vi "基恩士扫码枪.vi"(8 "error in":errorcluster) -> (0 "error out":errorcluster, 1 "扫码内容":string, 2 "扫码成功":bool)   [LabVIEW 2014]
uses:
  Controls/MsgAction.ctl
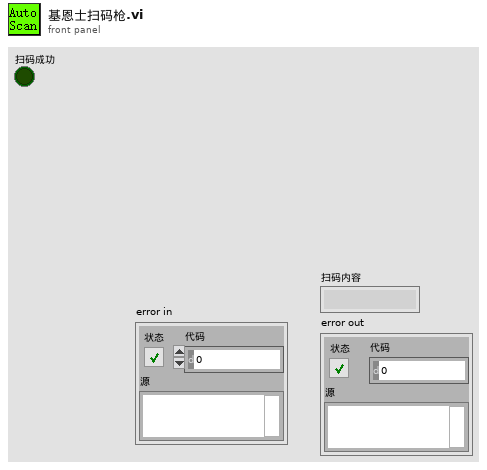
[diagram p1: front panel]
types:
  T1 = typedef "MsgAction.ctl" = enum16{"初始化", "添加消息", "区分结果添加消息", "清空消息", "获取消息"}
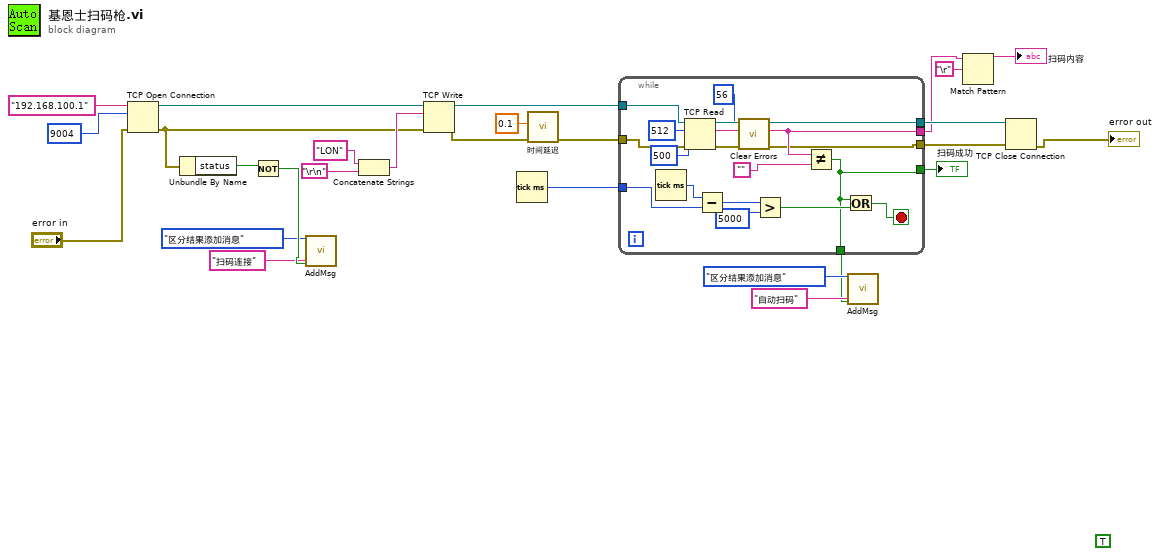
[diagram p0: block diagram]
diagram:
  (unwired) TRUE
  n1 = TCP Open Connection(address="192.168.100.1" ("地址"), remote port or service name=u16 9004 ("远程端口或服务名称"), error in (no error)="error in") -> (connection ID=w11:refnum<k5>, error out=w9:errorcluster)  [unwired: 2 in]
  n2 = Unbundle By Name(w9) -> ("status"=w26:bool)
  n3 = Not(x=w26) -> (.not. x?=w27:bool)
  n4 = call "AddMsg.vi"("Result"=w27, "添加消息"="扫码连接", "消息Action"=MsgAction."区分结果添加消息") -> ()  [unwired: 1 in, 1 out]
  n5 = Concatenate Strings("LON", "\r\n") -> (w19:string)
  n6 = TCP Write(connection ID=w11, data in=w19, error in (no error)=w9) -> (connection ID out=w18:refnum<k5>, error out=w14:errorcluster)  [unwired: 1 in, 1 out]
  n7 = Tick Count (ms)() -> (millisecond timer value=w5:u32)
  n8 = call "时间延迟"("error in (no error)"=w14, "Delay Time (s)"=0.1) -> ("error out"=w13:errorcluster)  [unwired: 9 in]
  n9 = while {
    tunnel: w18 -> [w44]
    tunnel: w13 -> [w42]
    tunnel: [w39] -> w8
    tunnel: [w31] -> w7
    tunnel: [w32] -> w3
    tunnel: [w28] -> w15
    tunnel: w5 -> [w29]
    tunnel: [w28] -> w4
    stop <- w34 stop-if-true
    n10 = Tick Count (ms)() -> (millisecond timer value=w40:u32)
    n11 = TCP Read(connection ID=w44, bytes to read=512 ("读取的字节"), error in (no error)=w42, 9:500 ("超时毫秒(25000)")) -> (connection ID out=w39:refnum<k5>, data out=w32:string, error out=w38:errorcluster)  [unwired: 1 in]
    n12 = Subtract(x=w40, y=w29) -> (x-y=w37:u32)
    n13 = call <vilib>:"Clear Errors.vi"("error in (no error)"=w38, "specific error code to clear (0: all)"=56) -> ("error out"=w31:errorcluster)  [unwired: 4 in, 1 out]
    n14 = Greater?(x=w37, y=u32 5000) -> (0:w35:bool)
    n15 = Not Equal?(x=w32, y="") -> (x != y?=w28:bool)
    n16 = Or(x=w28, y=w35) -> (x .or. y?=w34:bool)
  }
  "扫码成功" <- w4
  n17 = call "AddMsg.vi"("Result"=w15, "添加消息"="自动扫码", "消息Action"=MsgAction."区分结果添加消息") -> ()  [unwired: 1 in, 1 out]
  n18 = Match Pattern(string=w3, regular expression="\r") -> (before substring=→"扫码内容":string)  [unwired: 1 in, 3 out]
  n19 = TCP Close Connection(connection ID=w8, error in (no error)=w7) -> (error out=→"error out":errorcluster)  [unwired: 1 in, 1 out]
